vi "LINX SPI Benchmark.vi"(0 "Stop Button":bool) -> (3 "Loop Time (ms)":i32, 6 "Loop Rate":dbl(graph), 7 "Device Name":string)   [LabVIEW 2011]
uses:
  Private/Device/Device.lvlib
  Private/Type Defs/Interface.ctl
  LVH-LINX.lvlib
  <vilib>/ptbypt/NI_PtbyPt.lvlib
  Private/Type Defs/Peripherals/SPI/SPI CS Logic Level.ctl
panel:
  in  "CS Logic Level":T1
  in  "Frame Size":u8=1
  in  "CS Channel":u8=10
  out "Read Data":u8[](array[numeric])
  in  "Data":u8[](array[numeric]) format="%02x"
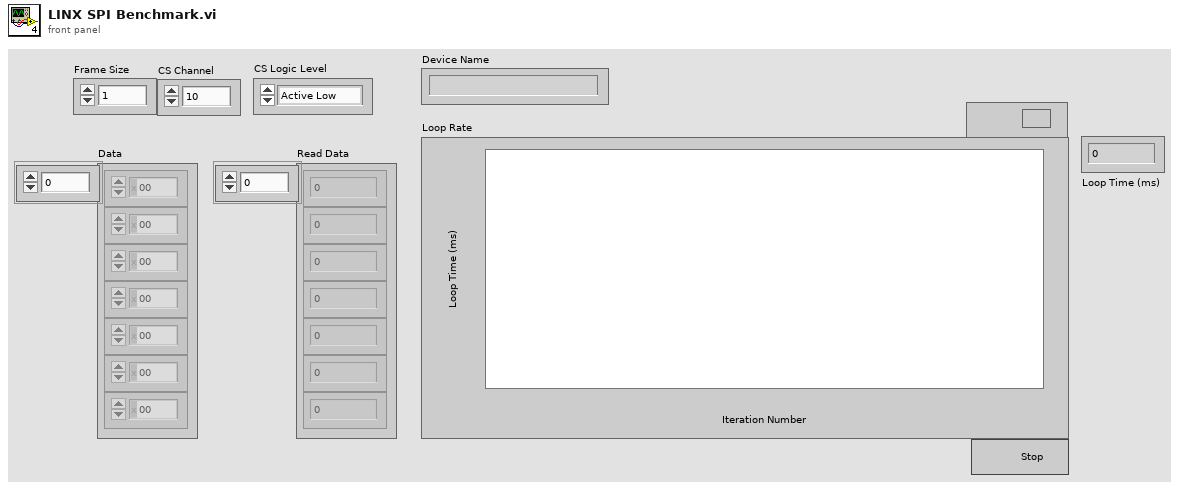
[diagram p1: front panel]
types:
  T1 = typedef "LVH-LINX.lvlib/SPI CS Logic Level.ctl" = enum8{"Active Low", "Active High"}
  T2 = typedef "LVH-LINX.lvlib/Interface.ctl" = enum16{"Serial", "TCP"}
  T3 = typedef "LVH-LINX.lvlib/Device.lvlib/LINX Device Config.ctl" = cluster{"Interface":T2, "COM Port":refnum<visa-resource-name>, "TCP Configuration":T4, "Device Family":T5, "Device ID":u8, "Device Name":string, "TCP Ref":refnum<k5>, "Channels":T6}
  T4 = typedef "LVH-LINX.lvlib/Device.lvlib/TCP Config.ctl" = cluster{"IP Address":string, "Port":u16}
  T5 = typedef "LVH-LINX.lvlib/Device Family.ctl" = enum8{"National Instruments", "Digilent", "Arduino"}
  T6 = typedef "LVH-LINX.lvlib/Channels.ctl" = cluster{"DI Channels":u8[], "DO Channels":u8[], "AI":u8[], "AO":u8[], "PWM":u8[], "QE":u8[], "UART":u8[], "I2C 2":u8[], "SPI":u8[], "CAN":u8[], "AI Ref (V)":dbl, "AO Resolution (Bits)":u8, "AO Ref (V)":dbl}
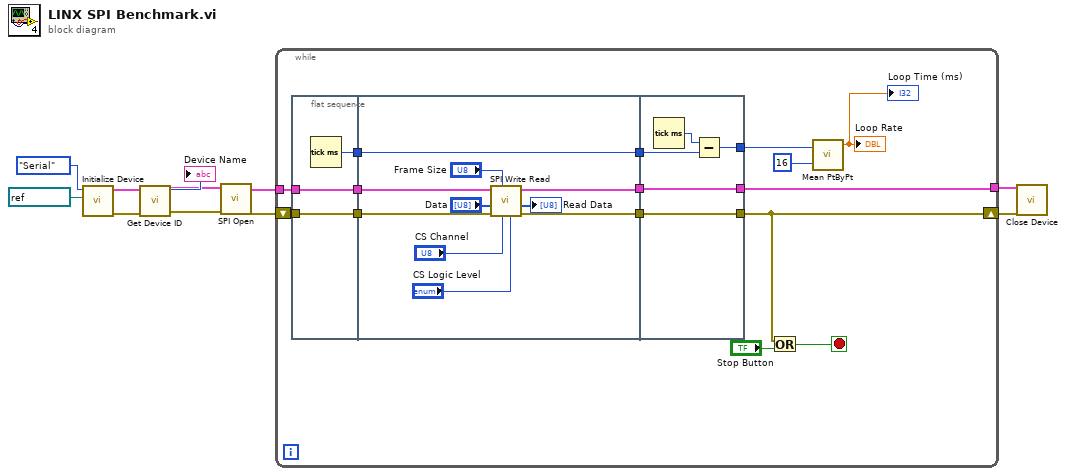
[diagram p0: block diagram]
diagram:
  n1 = call "Initialize Device.vi"("COM Port"=refnum<visa-resource-name> "COM5", "Interface"=Interface."Serial") -> ("Error Out"=w7:errorcluster, "LINX Device Config"=w8:T3)  [unwired: 8 in]
  n2 = call "Get Device ID.vi"("Error In"=w7, "LINX Device Config"=w8) -> ("Error Out"=w4:errorcluster, "Device Family"=→"Device Name":u8, "LINX Device Config"=w1:T3)  [unwired: 6 in, 1 out]
  n3 = call "SPI Open.vi"("Error In"=w4, "LINX Device Config"=w1) -> ("Error Out"=w3:errorcluster, "LINX Device Config"=w2:T3)  [unwired: 8 in]
  n4 = while {
    tunnel: w2 -> [w26]
    shift-right: [w12] -> w9
    shift-left: w3 -> [w14]
    tunnel: [w17] -> w5
    stop <- w25 stop-if-true
    n5 = flat-sequence {
      tunnel: w26 -> [w29]
      tunnel: [w29] -> w23
      tunnel: [w28] -> w22
      tunnel: w14 -> [w27]
      tunnel: [w27] -> w13
      tunnel: w23 -> [w35]
      tunnel: w22 -> [w39]
      tunnel: [w39] -> w21
      tunnel: [w38] -> w16
      tunnel: [w37] -> w15
      tunnel: w13 -> [w36]
      tunnel: w21 -> [w43]
      tunnel: [w42] -> w20
      tunnel: [w41] -> w17
      tunnel: w16 -> [w41]
      tunnel: w15 -> [w40]
      tunnel: [w40] -> w12
      frame #0 {
        n6 = Tick Count (ms)() -> (millisecond timer value=w28:u32)
      }
      frame #1 {
        n7 = call "SPI Write Read.vi"("CS Logic Level"="CS Logic Level", "CS Pin (10)"="CS Channel", "SPI Frame Size (1)"="Frame Size", "Error In"=w36, "Data"="Data", "LINX Device Config"=w35) -> ("Error Out"=w37:errorcluster, "Read Data"=→"Read Data":u8[], "LINX Device Config"=w38:T3)  [unwired: 3 in]
      }
      frame #2 {
        n8 = Tick Count (ms)() -> (millisecond timer value=w44:u32)
        n9 = Subtract(x=w44, y=w43) -> (x-y=w42:u32)
      }
    }
    n10 = Or(x=w12, y="Stop Button") -> (x .or. y?=w25:bool)
    n11 = call <vilib>:"Mean PtByPt.vi"("x"=w20, "sample length"=16) -> ("mean"=→"Loop Rate" →"Loop Time (ms)":dbl)  [unwired: 2 in, 1 out]
  }
  n12 = call "Close Device.vi"("Error In"=w9, "LINX Device Config"=w5) -> ()  [unwired: 8 in, 2 out]
